vi "Arm Teleop.vi"(9 "Slow Lift?":bool, 10 "Height Presets":T1, 11 "Speed":dbl) -> ()   [LabVIEW 2018]
panel:
  in  "Max dx/dt":dbl=3.0 format="%#_13g"
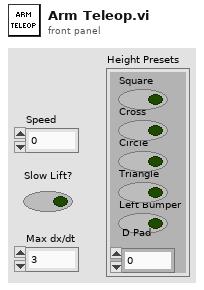
[diagram p1: front panel]
types:
  T1 = cluster{"Square":bool, "Cross":bool, "Circle":bool, "Triangle":bool, "Left Bumper":bool, "D Pad":i16}
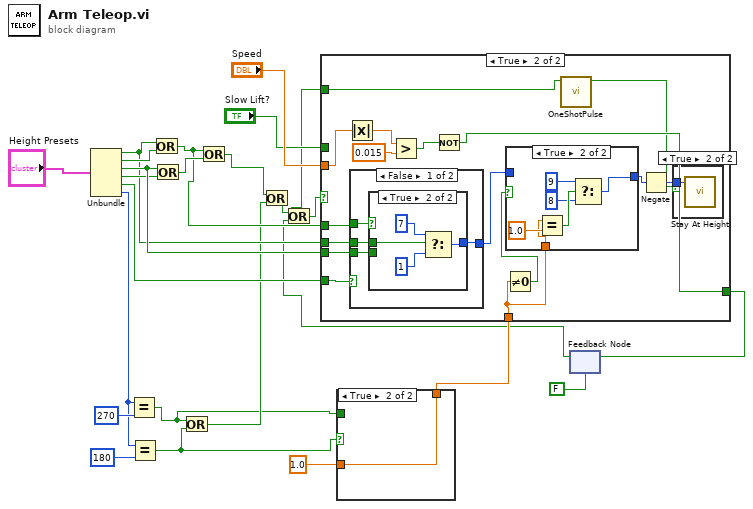
[diagram p0: block diagram]
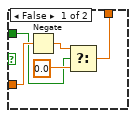
[diagram p2: hidden frame]
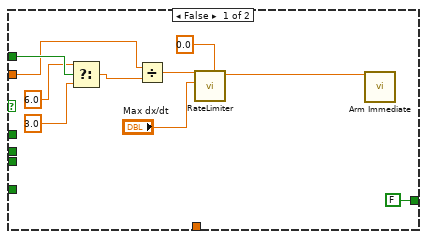
[diagram p3: hidden frame]
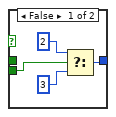
[diagram p6: hidden frame]
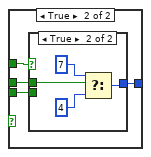
[diagram p7: hidden frame]
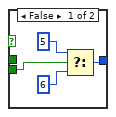
[diagram p8: hidden frame]
diagram:
  n1 = Unbundle("Height Presets") -> ("Square"=w12:bool, "Cross"=w23:bool, "Circle"=w22:bool, "Triangle"=w21:bool, "Left Bumper"=w18:bool, "D Pad"=w4:i16)
  n2 = Equal?(x=w4, y=270) -> (x = y?=w1:bool)
  n3 = Equal?(x=w4, y=180) -> (x = y?=w2:bool)
  n4 = Or(x=w12, y=w23) -> (x .or. y?=w13:bool)
  n5 = Or(x=w22, y=w21) -> (x .or. y?=w19:bool)
  n6 = Or(x=w1, y=w2) -> (x .or. y?=w3:bool)
  n7 = Or(x=w13, y=w19) -> (x .or. y?=w16:bool)
  n8 = Or(x=w16, y=w3) -> (x .or. y?=w7:bool)
  n9 = case shown="True" w2 {
    tunnel: [w26 w30] -> w14
    tunnel: 1.0 -> [w27 w30]
    tunnel: w1 -> [w25 _]
    frame False {
      n10 = Negate(x=w27) -> (-x=w28:dbl)
      n11 = Select(t=w28, s=w25, f=0.0) -> (s? t:f=w26:dbl)
    }
    frame True {
    }
  }
  n12 = feedback #1(FALSE) -> (w9:bool)
  n13 = Or(x=w7, y=w9) -> (x .or. y?=w10:bool)
  n14 = case shown="True" w10 {
    tunnel: "Speed" -> [w39 w47]
    tunnel: w13 -> [_ w56]
    tunnel: w22 -> [_ w55]
    tunnel: w18 -> [_ w54]
    tunnel: "Slow Lift?" -> [w40 _]
    tunnel: w14 -> [_ w50]
    tunnel: w12 -> [_ w49]
    tunnel: [FALSE w43] -> w8
    tunnel: w7 -> [_ w42]
    frame False {
      n15 = Select(t=6.0, s=w40, f=3.0) -> (s? t:f=w36:dbl)
      n16 = Divide(x=w39, y=w36) -> (x/y=w35:dbl)
      n17 = call "RateLimiter.vi"("Starting Value"=0.0, "Max dx/dt"="Max dx/dt", "Input"=w35) -> ("Output"=w32:dbl)  [unwired: 8 in]
      n18 = call "Arm Immediate.vi"("Speed"=w32) -> ()  [unwired: 10 in, 1 out]
    }
    frame True {
      n19 = Absolute Value(x=w47) -> (abs(x)=w46:dbl)
      n20 = case shown="False" w54 {
        tunnel: w56 -> [w68 w80]
        tunnel: [w66 w78] -> w53
        tunnel: w55 -> [w67 w79]
        tunnel: w49 -> [w65 w77]
        frame False {
          n21 = case shown="True" w68 {
            tunnel: [w71 w76] -> w66
            tunnel: w67 -> [w72 _]
            tunnel: w65 -> [_ w73]
            frame False {
              n22 = Select(t=2, s=w72, f=3) -> (s? t:f=w71:i32)
            }
            frame True {
              n23 = Select(t=7, s=w73, f=1) -> (s? t:f=w76:i32)
            }
          }
        }
        frame True {
          n24 = case shown="True" w80 {
            tunnel: [w83 w88] -> w78
            tunnel: w79 -> [w84 _]
            tunnel: w77 -> [_ w85]
            frame False {
              n25 = Select(t=5, s=w84, f=6) -> (s? t:f=w83:i32)
            }
            frame True {
              n26 = Select(t=7, s=w85, f=4) -> (s? t:f=w88:i32)
            }
          }
        }
      }
      n27 = Greater?(x=w46, y=0.015) -> (0:w44:bool)
      n28 = Not(x=w44) -> (.not. x?=w43:bool)
      n29 = Not Equal To 0?(x=w50) -> (x != 0?=w51:bool)
      n30 = case shown="True" w51 {
        tunnel: [w58 w59] -> w52
        tunnel: w53 -> [w58 _]
        tunnel: w50 -> [_ w63]
        frame False {
        }
        frame True {
          n31 = Equal?(x=w63, y=1.0) -> (x = y?=w62:bool)
          n32 = Select(t=i16 9, s=w62, f=i16 8) -> (s? t:f=w59:i16)
        }
      }
      n33 = call "OneShotPulse.vi"("Input"=w42) -> ("Output"=w41:bool)  [unwired: 10 in]
      n34 = Negate(x=w52) -> (-x=w48:i32)
      n35 = case shown="True" w41 {
        tunnel: w48 -> [_ w57]
        frame False {
        }
        frame True {
          n36 = call "Stay At Height.vi"("Height"=w57) -> ()  [unwired: 10 in, 1 out]
        }
      }
    }
  }
  n37 = feedback-in #1(w8) -> ()
